vi "ReturnName.vi"(8 "error in (no error)":errorcluster, 11 "Class in":refnum<class "Class.lvclass">) -> (0 "error out":errorcluster, 2 "Name":string, 3 "Class out":refnum<class "Class.lvclass">)   [LabVIEW 2020, in "Mermaid.lvlib" / "Class.lvclass"]
uses:
  Class.lvclass
  Class.lvclass/Class.ctl
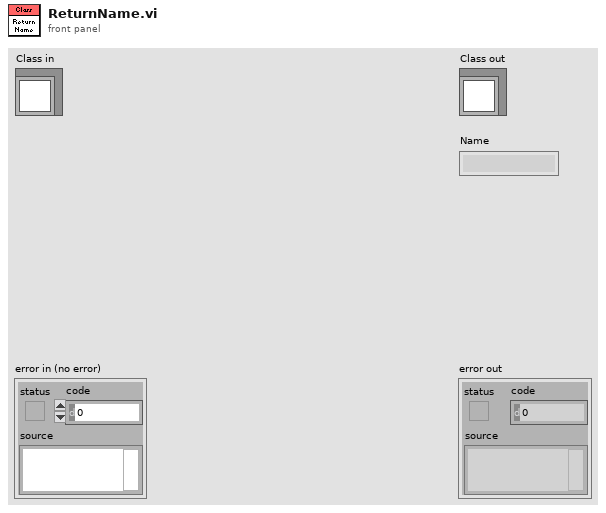
[diagram p1: front panel]
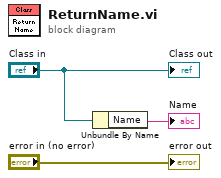
[diagram p0: block diagram]
diagram:
  n1 = Unbundle By Name("Class in") -> ("Name"=→"Name":string)
  "error out" <- "error in (no error)"
  "Class out" <- "Class in"
